vi "(SubVI) 2D-Gaussian Fit image.vi"(8 "error in (no error)":errorcluster, 10 "initial parameters":dbl[](array[numeric])=[100.0, 3.0, 3.0, 10.0, 10.0, 0.0, 8.0], 11 "Input Image":T1(plugin-control)) -> (0 "error out":errorcluster, 1 "best fit parameters":dbl[](array[numeric]), 2 "y position (nm)":dbl, 3 "x position (nm)":dbl)   [LabVIEW 2014]
uses:
  <vilib>/gmath/NumericalOptimization/Nonlinear Curve Fit LM.vi
  <vilib>/gmath/NI_Gmath.lvlib
panel:
  out "image size(pixel)":i32
  out "cf (nm/pixel)":dbl
  # "A, \nsx, \nsy, \nx0, \ny0, \ntheta(deg), \noffset"
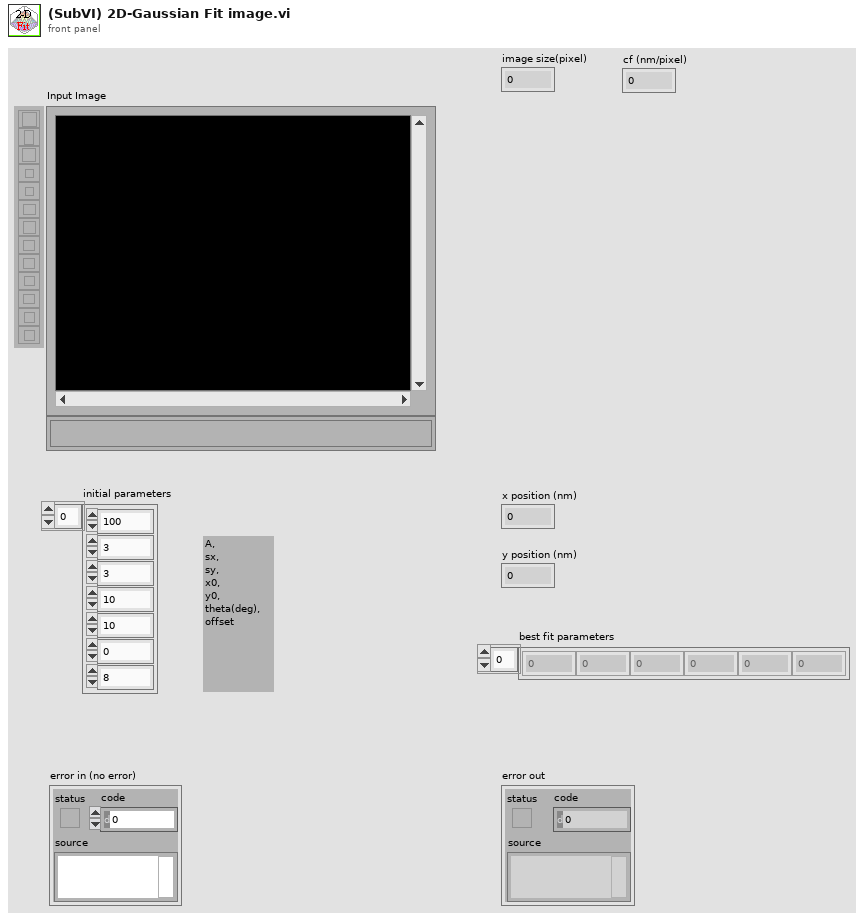
[diagram p1: front panel]
types:
  T1 = typedef "IMAQ Image.ctl" = refnum<image>
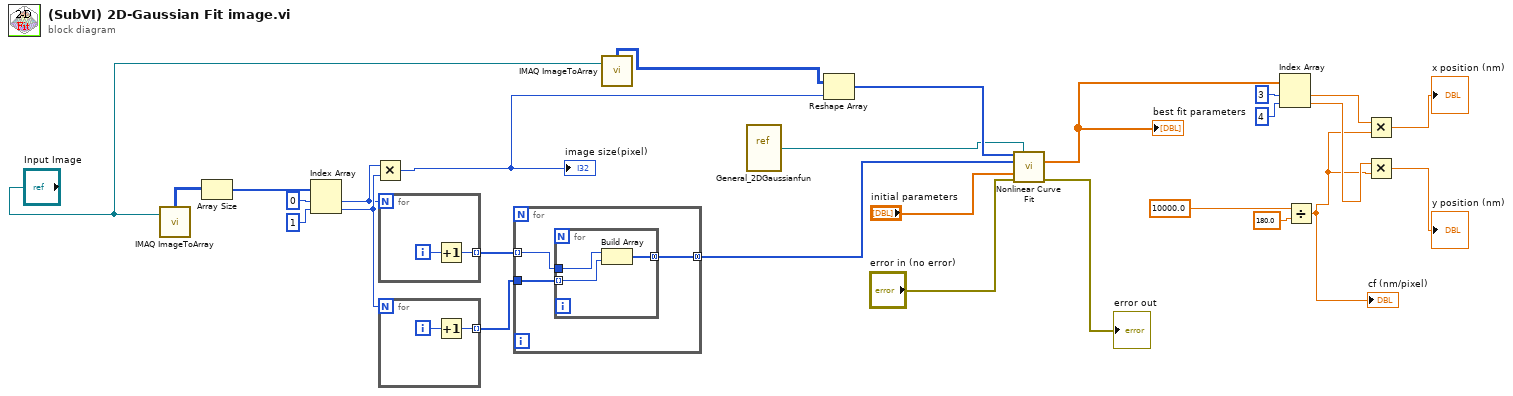
[diagram p0: block diagram]
diagram:
  n1 = call "IMAQ ImageToArray"("Image"="Input Image") -> ("Image Pixels (U8)"=w16:u8[][])  [unwired: 3 in, 4 out]
  n2 = Array Size(array=w16) -> (size(s)=w17:i32[])
  n3 = Index Array(array=w17, index #1=0 ("index"), index #2=1 ("index")) -> (element #1=w18:i32, element #2=w19:i32)
  n4 = Multiply(x=w18, y=w19) -> (x*y=w2:i32)
  "image size(pixel)" <- w2
  n5 = for {
    N: w18 -> [_]
    tunnel: [w28] -> w20 mode=indexing
    i -> [w29]
    n6 = Increment(x=w29) -> (x+1=w28:i32)
  }
  n7 = for {
    N: w19 -> [_]
    tunnel: [w30] -> w21 mode=indexing
    i -> [w31]
    n8 = Increment(x=w31) -> (x+1=w30:i32)
  }
  n9 = for {
    tunnel: w20 -> [w34] mode=indexing
    tunnel: w21 -> [w33]
    tunnel: [w32] -> w3 mode=concatenating
    n10 = for {
      tunnel: w34 -> [w36]
      tunnel: w33 -> [w35] mode=indexing
      tunnel: [w37] -> w32 mode=concatenating
      n11 = Build Array(w36, w35) -> (w37:i32[])
    }
  }
  n12 = call "IMAQ ImageToArray"("Image"="Input Image") -> ("Image Pixels (U8)"=w6:u8[][])  [unwired: 3 in, 4 out]
  n13 = vi-ref "General_2DGaussianfun.vi"() -> (w1:refnum<vi>)
  n14 = Reshape Array(w6, w2) -> (w11:u8[])
  n15 = call-poly <vilib>:"Nonlinear Curve Fit.vi"("Y"=w11, "f(x,a)"=w1, "X"=w3, "initial parameters"="initial parameters", "error in (no error)"="error in (no error)") -> ("best fit parameters"=w8:dbl[], "error out"=→"error out":errorcluster)  [unwired: 5 in, 4 out]
  "best fit parameters" <- w8
  n16 = Index Array(array=w8, index #1=3 ("index"), index #2=4 ("index")) -> (element #1=w22:dbl, element #2=w25:dbl)
  n17 = Divide(x=10000.0, y=180.0) -> (x/y=w24:dbl)
  "cf (nm/pixel)" <- w24
  n18 = Multiply(x=w22, y=w24) -> (x*y=→"x position (nm)":dbl)
  n19 = Multiply(x=w25, y=w24) -> (x*y=→"y position (nm)":dbl)
